vi "Range_selector.vi"(8 "potential":dbl, 11 "current":dbl) -> (3 "range integer":i32)   [LabVIEW 2022 SP3]
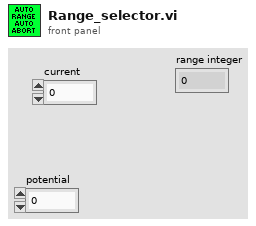
[diagram p1: front panel]
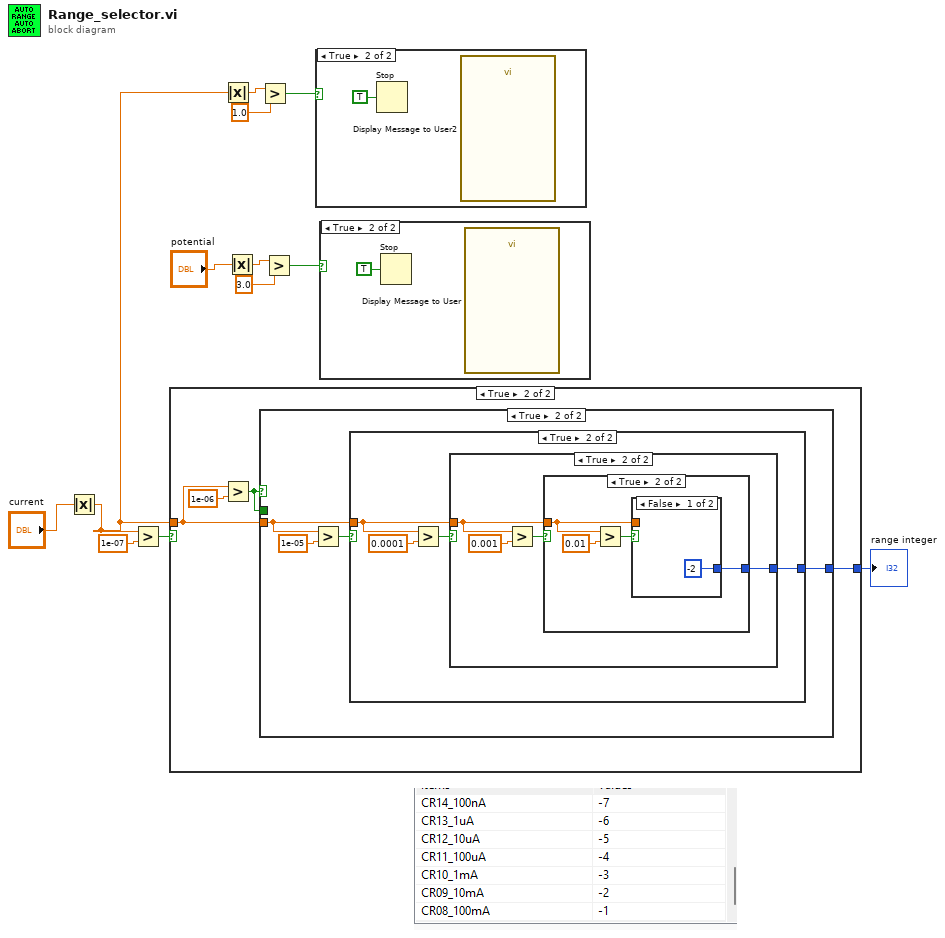
[diagram p0: block diagram]
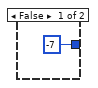
[diagram p4: hidden frame]
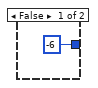
[diagram p5: hidden frame]
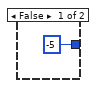
[diagram p6: hidden frame]
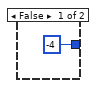
[diagram p7: hidden frame]
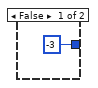
[diagram p8: hidden frame]
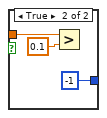
[diagram p9: hidden frame]
diagram:
  n1 = Absolute Value(x="current") -> (abs(x)=w1:dbl)
  n2 = Greater?(x=w1, y=1e-07) -> (0:w11:bool)
  n3 = case shown="True" w11 {
    tunnel: w1 -> [_ w16]
    tunnel: [-7 w14] -> w10
    frame False {
    }
    frame True {
      n4 = Greater?(x=w16, y=1e-06) -> (0:w15:bool)
      n5 = case shown="True" w15 {
        tunnel: w15 -> [_ _]
        tunnel: w16 -> [_ w20]
        tunnel: [-6 w19] -> w14
        frame False {
        }
        frame True {
          n6 = Greater?(x=w20, y=1e-05) -> (0:w21:bool)
          n7 = case shown="True" w21 {
            tunnel: w20 -> [_ w25]
            tunnel: [-5 w24] -> w19
            frame False {
            }
            frame True {
              n8 = Greater?(x=w25, y=0.0001) -> (0:w26:bool)
              n9 = case shown="True" w26 {
                tunnel: w25 -> [_ w30]
                tunnel: [-4 w29] -> w24
                frame False {
                }
                frame True {
                  n10 = Greater?(x=w30, y=0.001) -> (0:w31:bool)
                  n11 = case shown="True" w31 {
                    tunnel: w30 -> [_ w35]
                    tunnel: [-3 w34] -> w29
                    frame False {
                    }
                    frame True {
                      n12 = Greater?(x=w35, y=0.01) -> (0:w36:bool)
                      n13 = case shown="False" w36 {
                        tunnel: w35 -> [_ w40]
                        tunnel: [-2 -1] -> w34
                        frame False {
                        }
                        frame True {
                          n14 = Greater?(x=w40, y=0.1) -> ()  [unwired: 1 out]
                        }
                      }
                    }
                  }
                }
              }
            }
          }
        }
      }
    }
  }
  "range integer" <- w10
  n15 = Absolute Value(x=w1) -> (abs(x)=w6:dbl)
  n16 = Absolute Value(x="potential") -> (abs(x)=w8:dbl)
  n17 = Greater?(x=w6, y=1.0) -> (0:w3:bool)
  n18 = Greater?(x=w8, y=3.0) -> (0:w4:bool)
  n19 = case shown="True" w3 {
    frame False {
    }
    frame True {
      n20 = Stop(stop? (T)=TRUE) -> ()
      n21 = call "Display Message to User2"() -> ()  [unwired: 10 in, 2 out]
    }
  }
  n22 = case shown="True" w4 {
    frame False {
    }
    frame True {
      n23 = Stop(stop? (T)=TRUE) -> ()
      n24 = call "Display Message to User"() -> ()  [unwired: 10 in, 2 out]
    }
  }
